vi "Item Add.vi"(0 "Tree Reference In":refnum<vi>, 1 "Parent Tag (Current)":string, 2 "New Tag Value (Same as Text)":string, 3 "New Text Value":string, 5 "error in (no error)":errorcluster, 6 "Child Only?":bool, 8 "Make Top Level Item":bool, 9 "Column Text{#1 and greater}(empty)":string[](array[string])) -> (14 "Tree Reference Out":refnum<vi>, 16 "Created Tag":string, 19 "error out":errorcluster)   [LabVIEW 2014]
doc: "Adds a new item to the tree. Uses the current selection if there is no parent value input. The tag is set to the same value as the input text if it is left blank. NOTE: TAGS MUST BE UNIQUE."
panel:
  # "VI INPUTS"
  # "VI OUTPUTS"
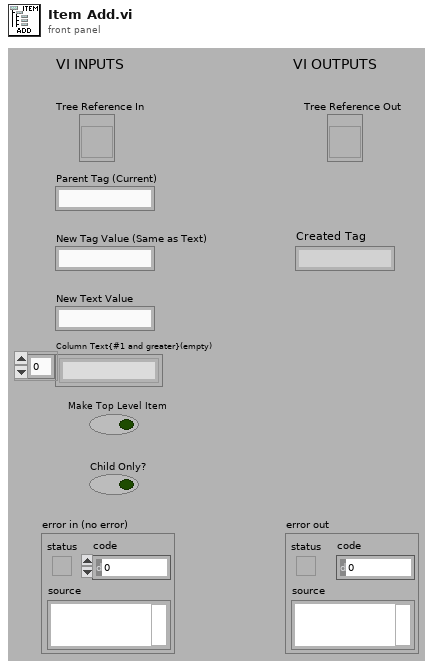
[diagram p1: front panel]
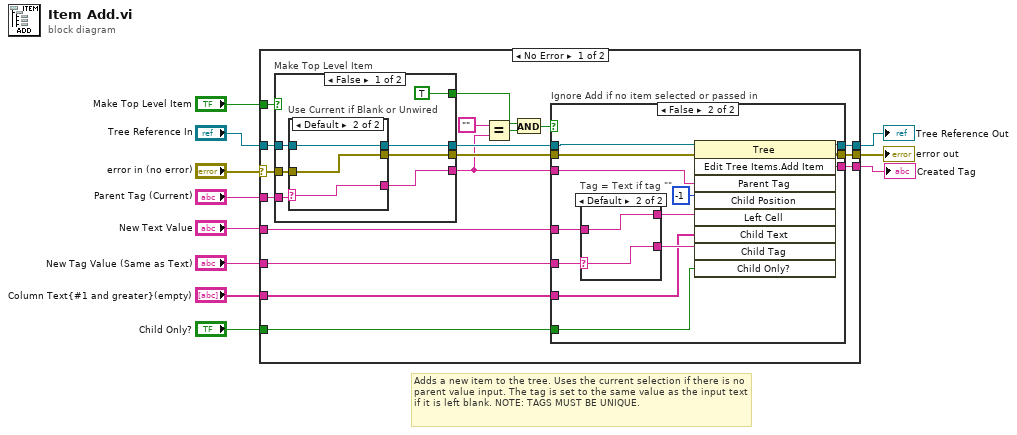
[diagram p0: block diagram]
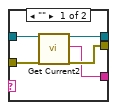
[diagram p2: hidden frame]
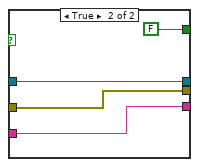
[diagram p3: hidden frame]
diagram:
  # "Adds a new item to the tree. Uses the current selection if there is no parent value input. The tag is set to the same value as the input text if it is left blank. NOTE: TAGS MUST BE UNIQUE."
  n1 = case shown="No Error" "error in (no error)" {
    selector: "error in (no error)" -> [w27 w69]
    tunnel: "Tree Reference In" -> [w29 w70]
    tunnel: [w26 w70] -> w10
    tunnel: [w25 w69] -> w9
    tunnel: "Parent Tag (Current)" -> [w28 w68]
    tunnel: "New Text Value" -> [w22 _]
    tunnel: "New Tag Value (Same as Text)" -> [w21 _]
    tunnel: "Column Text{#1 and greater}(empty)" -> [w20 _]
    tunnel: "Make Top Level Item" -> [w19 _]
    tunnel: "Child Only?" -> [w13 _]
    tunnel: [w12 w68] -> w1
    frame No Error {
      n2 = case "Make Top Level Item" shown="False" w19 {
        tunnel: w29 -> [w36 w48]
        tunnel: w28 -> [w35 w46]
        tunnel: w27 -> [w34 w47]
        tunnel: [w33 w48] -> w24
        tunnel: [w32 w47] -> w23
        tunnel: [w31 w46] -> w15
        tunnel: [TRUE FALSE] -> w16
        frame False {
          n3 = case "Use Current if Blank or Unwired" shown="Default" w35 {
            selector: w35 -> [_ w42]
            tunnel: [w40 w44] -> w33
            tunnel: w36 -> [w41 w44]
            tunnel: [w39 w43] -> w32
            tunnel: w34 -> [w38 w43]
            tunnel: [w37 w42] -> w31
            frame "" {
              n4 = call "Get Current2.vi"("Tree Reference In"=w41, "error in (no error)"=w38) -> ("Tree Reference Out"=w40:refnum<vi>, "Current Tag"=w37:string, "error out"=w39:errorcluster)  [unwired: 14 in, 1 out]
            }
            frame Default {
            }
          }
        }
        frame True {
        }
      }
      n5 = Equal?(x="", y=w15) -> (x = y?=w17:bool)
      n6 = And(x=w16, y=w17) -> (x .and. y?=w14:bool)
      n7 = case "Ignore Add if no item selected or passed in" shown="False" w14 {
        tunnel: [w51 w58] -> w26
        tunnel: [w50 w57] -> w25
        tunnel: w24 -> [w51 w62]
        tunnel: w23 -> [w50 w61]
        tunnel: w22 -> [_ w63]
        tunnel: w21 -> [_ w64]
        tunnel: w20 -> [_ w56]
        tunnel: w15 -> [w49 w55]
        tunnel: w13 -> [_ w54]
        tunnel: [w49 w53] -> w12
        frame True {
        }
        frame False {
          n8 = case "Tag = Text if tag \"\"" shown="Default" w64 {
            selector: w64 -> [_ w66]
            tunnel: w63 -> [w65 w67]
            tunnel: [w65 w67] -> w60
            tunnel: [w65 w66] -> w59
            frame "" {
            }
            frame Default {
            }
          }
          n9 = invoke class="Tree" method="Edit Tree Items.Add Item"(reference=w62, error in=w61, "Parent Tag"=w55, "Child Position"=-1, "Left Cell"=w60, "Child Text"=w56, "Child Tag"=w59, "Child Only?"=w54) -> (reference out=w58:refnum<vi>, error out=w57:errorcluster, "Edit Tree Items:Add Item"=w53:string)  [unwired: 1 in, 6 out]
        }
      }
    }
    frame Error {
    }
  }
  "Tree Reference Out" <- w10
  "error out" <- w9
  "Created Tag" <- w1
